vi "Insert Subpanel.vi"(6 "Page Refnum":refnum<vi>, 8 "error in (no error)":errorcluster, 9 "Subpanel reference":refnum<vi>, 10 "node References":T7, 11 "References":T1) -> (0 "error out":errorcluster)   [LabVIEW 2015, in "E2E Tag Exchange editor node.lvclass"]
uses:
  E2E Tag Exchange editor node.lvclass
  object references.ctl
  <vilib>/NI/DCAF/Tag Editor Core/Configuration Editor/Classes/Engine Parent/Engine Parent Editor Node.lvclass
  references.ctl
  <vilib>/NI/Configuration Framework/Node/StopEvent.ctl
  <vilib>/NI/Configuration Framework/Node/RefreshUIEvent.ctl
  <vilib>/NI/Configuration Framework/Node/CacheState.ctl
  <vilib>/NI/Configuration Framework/Node/NodeChangeEvent.ctl
  <vilib>/NI/Configuration Framework/Node/NodeRef.ctl
  <vilib>/NI/Configuration Framework/Node/NISE_CEF_Node.lvclass
  <vilib>/NI/AMC/Message Queue.ctl
  <vilib>/NI/AMC/Message.ctl
  <vilib>/NI/Tools/Keyed Array/KeyedArray.ctl
  <vilib>/NI/Tools/Keyed Array/Tools_KeyedArray.lvlib
  <vilib>/NI/AMC/AMC.lvlib
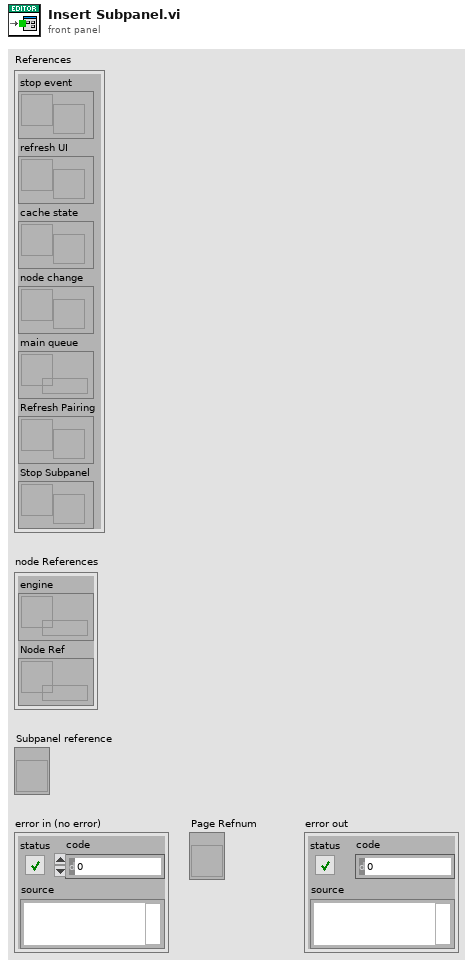
[diagram p1: front panel]
types:
  T1 = typedef "E2E Tag Exchange editor node.lvclass/references.ctl" = cluster{"stop event":T2, "refresh UI":T3, "cache state":T4, "node change":T5, "main queue":T6, "Refresh Pairing":refnum<user-event>, "Stop Subpanel":refnum<user-event>}
  T2 = typedef "NISE_CEF_Node.lvclass/StopEvent.ctl" = refnum<user-event>
  T3 = typedef "NISE_CEF_Node.lvclass/RefreshUIEvent.ctl" = refnum<user-event>
  T4 = typedef "NISE_CEF_Node.lvclass/CacheState.ctl" = refnum<user-event>
  T5 = typedef "NISE_CEF_Node.lvclass/NodeChangeEvent.ctl" = refnum<user-event>
  T6 = typedef "AMC.lvlib/Message Queue.ctl" = refnum<queue>
  T7 = typedef "E2E Tag Exchange editor node.lvclass/object references.ctl" = cluster{"engine":refnum<data-value>, "Node Ref":refnum<data-value>}
  T8 = typedef "E2E Tag Exchange configuration.lvclass/Runtime Implementation.ctl" = enum16{"RT FIFO", "UDP"}
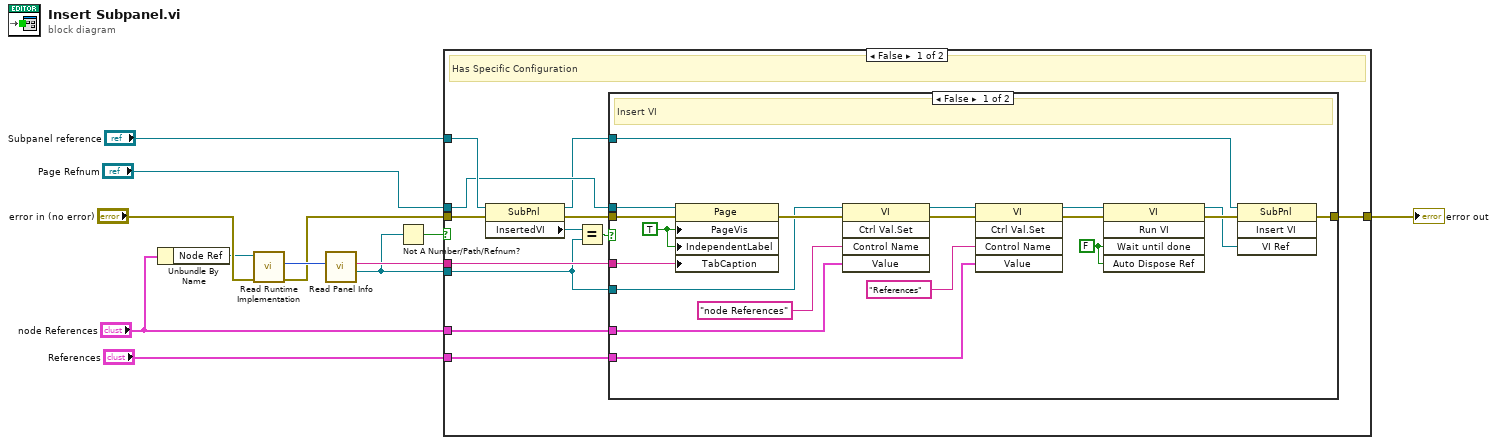
[diagram p0: block diagram]
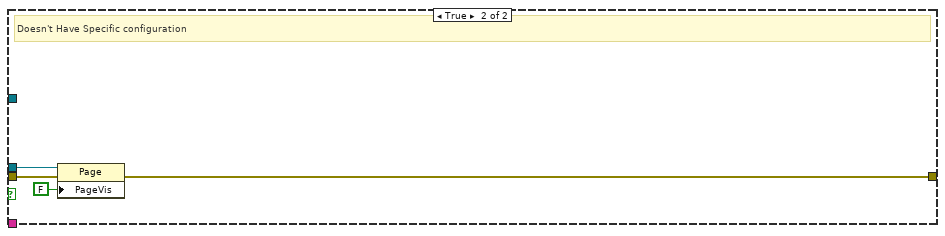
[diagram p3: hidden frame]
diagram:
  n1 = Unbundle By Name("node References") -> ("Node Ref"=w6:refnum<data-value>)
  n2 = call "Read Runtime Implementation.vi"("error in (no error)"="error in (no error)", "E2E editor node in"=w6) -> ("error out"=w1:errorcluster, "Runtime Implementation"=w8:T8)  [unwired: 7 in, 1 out]
  n3 = call "Read Panel Info.vi"("Runtime Implementation"=w8) -> ("VI Refnum"=w2:refnum<vi>, "Tab Name"=w11:string)  [unwired: 9 in]
  n4 = Not A Number/Path/Refnum?(number/path/refnum=w2) -> (NaN/Path/Refnum?=w3:bool)
  n5 = case shown="False" w3 {
    tunnel: "Page Refnum" -> [w19 w48]
    tunnel: w11 -> [w24 _]
    tunnel: "node References" -> [w23 _]
    tunnel: "References" -> [w22 _]
    tunnel: [w21 w45] -> w9
    tunnel: w2 -> [w14 _]
    tunnel: w1 -> [w18 w47]
    tunnel: "Subpanel reference" -> [w20 _]
    frame False {
      # "Has Specific Configuration"
      n6 = property class="SubPnl"(reference=w20, error in=w18) -> (reference out=w13:refnum<vi>, error out=w17:errorcluster, "InsertedVI"=w16:refnum<vi>)
      n7 = Equal?(x=w16, y=w14) -> (x = y?=w15:bool)
      n8 = case shown="False" w15 {
        tunnel: w19 -> [w43 _]
        tunnel: w24 -> [w41 _]
        tunnel: w14 -> [w39 _]
        tunnel: w23 -> [w38 _]
        tunnel: w22 -> [w34 _]
        tunnel: [w27 w44] -> w21
        tunnel: w17 -> [w26 w44]
        tunnel: w13 -> [w25 _]
        frame False {
          w32 = FALSE ("Wait Until Done")
          w42 = TRUE ("Page Visible")
          # "Insert VI"
          n9 = property class="Page"(reference=w43, error in=w26, "PageVis"=w42, "IndependentLabel"=w42, "TabCaption"=w41) -> (error out=w40:errorcluster)  [unwired: 1 out]
          n10 = invoke class="VI" method="Ctrl Val.Set"(reference=w39, error in=w40, "Control Name"="node References", "Value"=w38) -> (reference out=w36:refnum<vi>, error out=w35:errorcluster)  [unwired: 1 in, 3 out]
          n11 = invoke class="VI" method="Ctrl Val.Set"(reference=w36, error in=w35, "Control Name"="References", "Value"=w34) -> (reference out=w29:refnum<vi>, error out=w28:errorcluster)  [unwired: 1 in, 3 out]
          n12 = invoke class="VI" method="Run VI"(reference=w29, error in=w28, "Wait until done"=w32, "Auto Dispose Ref"=w32) -> (reference out=w30:refnum<vi>, error out=w31:errorcluster)  [unwired: 1 in, 3 out]
          n13 = invoke class="SubPnl" method="Insert VI"(reference=w25, error in=w31, "VI Ref"=w30) -> (error out=w27:errorcluster)  [unwired: 1 in, 3 out]
        }
        frame True {
          # "VI Already Inserted"
        }
      }
    }
    frame True {
      # "Doesn't Have Specific configuration"
      n14 = property class="Page"(reference=w48, error in=w47, "PageVis"=FALSE ("Page Visible")) -> (error out=w45:errorcluster)  [unwired: 1 out]
    }
  }
  "error out" <- w9
